vi "LJUD_eGetPtrS (DBL Array).vi"(5 "Channel":i32, 7 "IOType":string, 8 "error in":errorcluster, 9 "DBL Array Write":dbl[](array[numeric]) format="%.2f", 10 "Value":i32, 11 "Handle In":i32) -> (0 "error out":errorcluster, 1 "DBL Array Read":dbl[](array[numeric]) format="%.2f", 2 "Value":i32, 3 "Handle Out":i32)   [LabVIEW 2021]
doc: "In this version of eGet the\nIOType is a string. This is a special\nLabVIEW variation of eGetS where\nx1 is declared as a DBL array.\n\nThis is a traditional technique UD\nfunction that internally performs\na single Add, a GoOne, and a single\nGet. See Section 4.1 of the device's\ndatasheet for more information.\n\nIOType specifies what sort of action\nwill be performed. The other inputs\ndepend on the IOType. See the\npseudocode in Section 4.3 for info."
uses:
  labjackud.dll
panel:
  # "For 32-bit and 64-bit support, this\nvariation uses eGetPtr rather\nthan eGet.\n\nIn this version of eGet the\nIOType is a string.  This is a special\nLabVIEW variation of eGetS where\nx1 is declared as a DBL array.\n\nThis is a traditional technique UD\nfunction that internally performs\na single Add, a GoOne, and a single\nGet.  See Section 4.1 of the device's\ndatasheet for more information.\n\nIOType specifies what sort of action\nwill be performed.  The other inputs\ndepend on the IOType.  See the\npseudocode in Section 4.3 for info."
  # "Uses \"Reentrant\" for the DLL call."
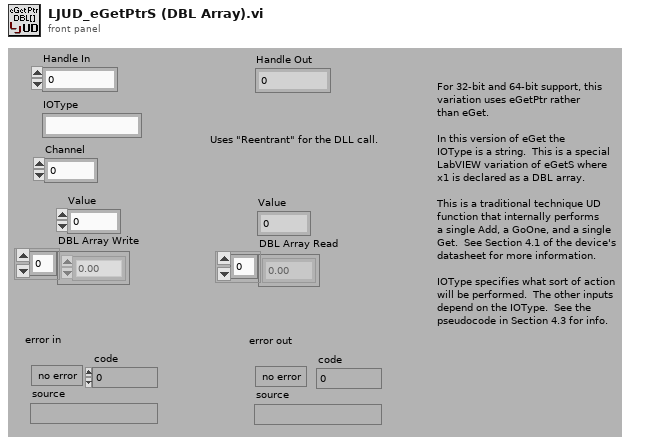
[diagram p1: front panel]
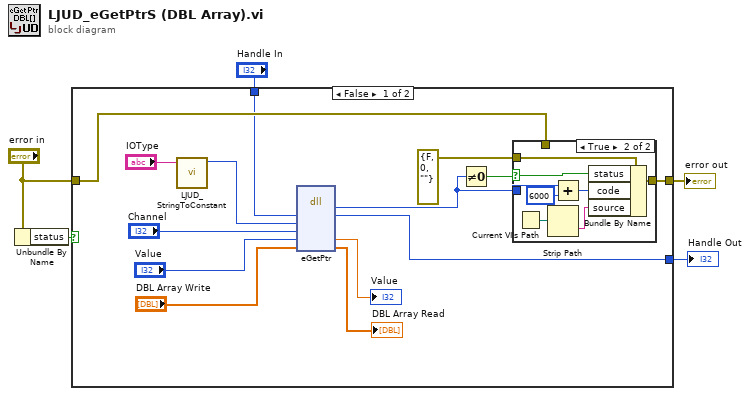
[diagram p0: block diagram]
diagram:
  n1 = Unbundle By Name("error in") -> ("status"=w4:bool)
  n2 = case shown="False" w4 {
    tunnel: [w14 w30] -> w5
    tunnel: "error in" -> [w10 w30]
    tunnel: "Handle In" -> [w9 w29]
    tunnel: [w8 w29] -> w1
    frame False {
      n3 = call "LJUD_StringToConstant.vi"("String"="IOType") -> ("Constant Number"=w6:i32)  [unwired: 9 in, 1 out]
      n4 = dll-call lib="labjackud.dll" fn="eGetPtr"("Handle"=w9, "IOType"=w6, "Channel"="Channel", "Value"="Value", "x1"="DBL Array Write") -> (w11:i32, "Handle"=w8:i32, "Value"=→"Value":dbl, "x1"=→"DBL Array Read":dbl[])  [unwired: 5 in, 2 out]
      n5 = Not Equal To 0?(x=w11) -> (x != 0?=w12:bool)
      n6 = case shown="True" w12 {
        selector: w12 -> [_ w27]
        tunnel: [w20 w28] -> w14
        tunnel: errorcluster {"status"=FALSE, "code"=0, "source"=""} ("error IO") -> [_ w26]
        tunnel: w11 -> [_ w22]
        tunnel: w10 -> [w20 _]
        frame False {
        }
        frame True {
          n7 = Current VI's Path() -> (path=w24:path)
          n8 = Strip Path(path=w24) -> (name=w25:string)  [unwired: 1 out]
          n9 = Add(x=w22, y=6000) -> (x+y=w23:i32)
          n10 = Bundle By Name(cluster=w26, "status"=w27, "code"=w23, "source"=w25) -> (w28:errorcluster)
        }
      }
    }
    frame True {
    }
  }
  "error out" <- w5
  "Handle Out" <- w1
